vi "Write.vi"(8 "error in (no error)":errorcluster, 10 "element":variant, 11 "NetworkStreamWriter in":refnum<class "NetworkStreamWriter.lvclass">) -> (0 "error out":errorcluster, 1 "Successful?":bool, 3 "NetworkStreamWriter out":refnum<class "NetworkStreamWriter.lvclass">)   [LabVIEW 2011, in "NetworkStreamWriter.lvclass"]
doc: "Returns the requested value (either the next element available in the buffer or the most recent element). If there are no elements available in the queue, this VI will return the last valid value it returned.\n\nWrites the requested value to the internal queue, which will be sent across the network asynchronously by the WriterDaemon."
uses:
  NetworkStreamWriter.lvclass
  NetworkStreamWriter.lvclass/NetworkStreamWriter.ctl
  Shared/message.ctl
panel:
  out "Initialized?":bool
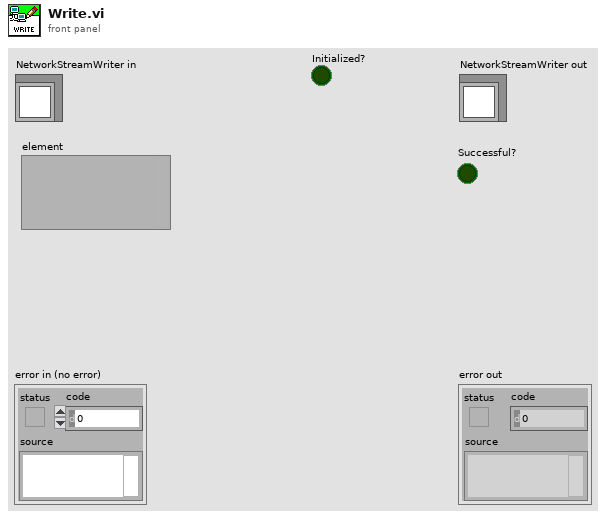
[diagram p1: front panel]
types:
  T1 = typedef "message.ctl" = cluster{"Data":variant, "Time since start (s)":dbl}
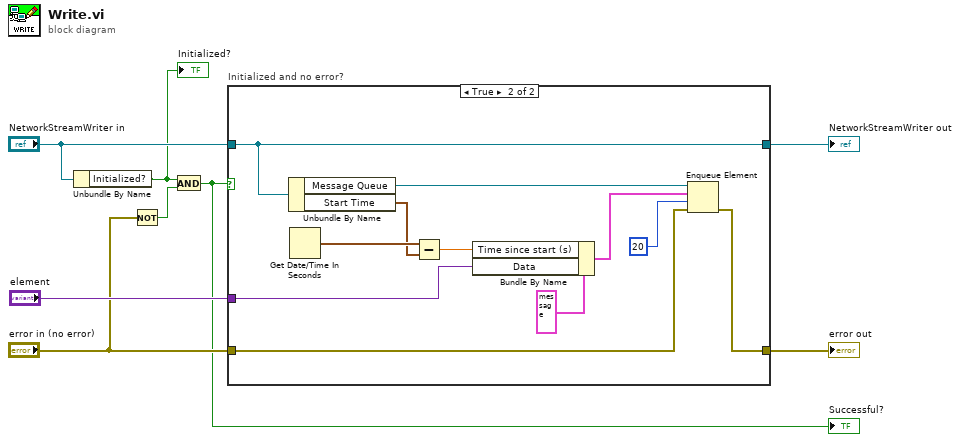
[diagram p0: block diagram]
diagram:
  n1 = Unbundle By Name("NetworkStreamWriter in") -> ("Initialized?"=w3:bool)
  "Initialized?" <- w3
  n2 = Not(x="error in (no error)") -> (.not. x?=w4:bool)
  n3 = And(x=w3, y=w4) -> (x .and. y?=w1:bool)
  "Successful?" <- w1
  n4 = case "Initialized and no error?" shown="True" w1 {
    tunnel: [w9 w18] -> w8
    tunnel: [w10 w21] -> w7
    tunnel: "NetworkStreamWriter in" -> [w10 w21]
    tunnel: "element" -> [_ w13]
    tunnel: "error in (no error)" -> [w9 w11]
    frame False {
    }
    frame True {
      n5 = Unbundle By Name(w21) -> ("Message Queue"=w20:refnum<queue>, "Start Time"=w16:timestamp)
      n6 = Get Date/Time In Seconds() -> (seconds since 1Jan1904=w17:timestamp)
      n7 = Subtract(x=w17, y=w16) -> (x-y=w14:dbl)
      n8 = Bundle By Name(cluster=T1 {"Data"=variant, "Time since start (s)"=0.0} ("Message"), "Time since start (s)"=w14, "Data"=w13) -> (w12:T1)
      n9 = Enqueue Element(queue=w20, element=w12, timeout in ms (-1)=20, error in (no error)=w11) -> (error out=w18:errorcluster)  [unwired: 2 out]
    }
  }
  "error out" <- w8
  "NetworkStreamWriter out" <- w7
